vi "CAN Log File Data Write.vi"(5 "Size":string, 7 "Socket":i16, 8 "error in (no error)":errorcluster, 9 "With Column and CAN Data":string, 10 "Without Column and CAN Data":string, 11 "Byte Stream File in":refnum<file>) -> (0 "error out":errorcluster, 3 "Byte Stream File out":refnum<file>)   [LabVIEW 2023, in "LTT_TeststandSteptypes.lvlib"]
uses:
  LTT_TeststandSteptypes.lvlib
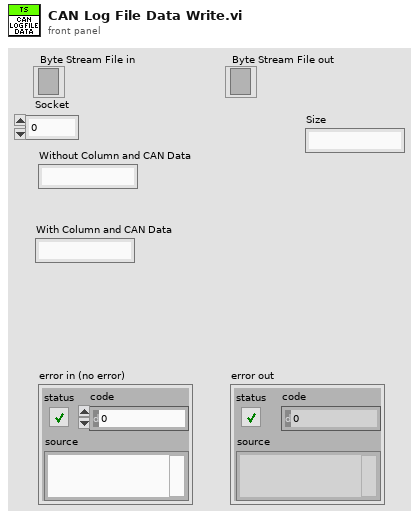
[diagram p1: front panel]
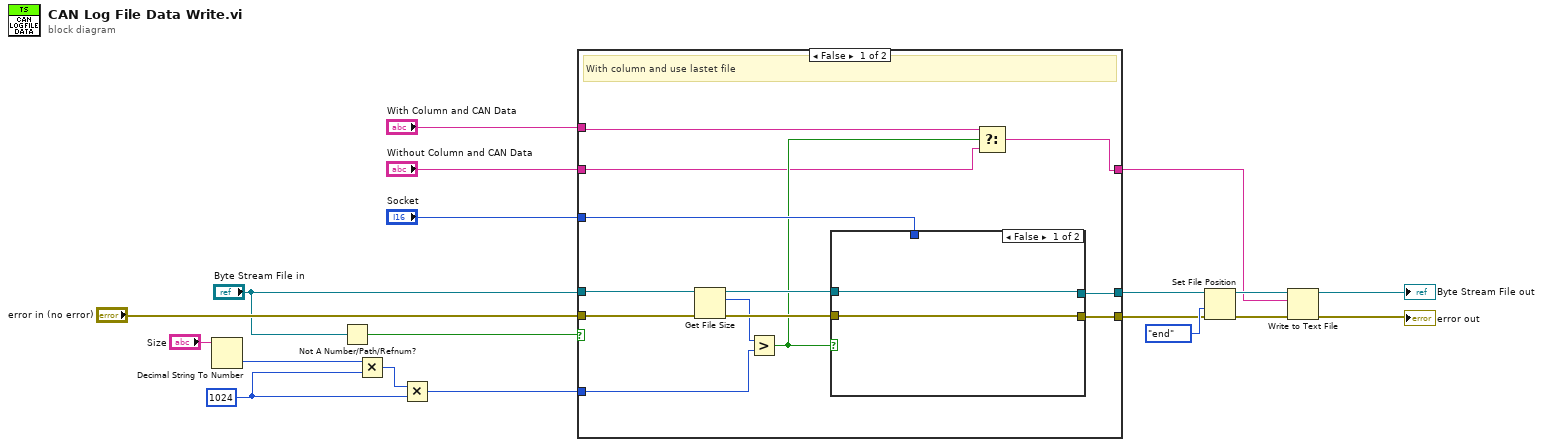
[diagram p0: block diagram]
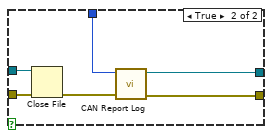
[diagram p2: hidden frame]
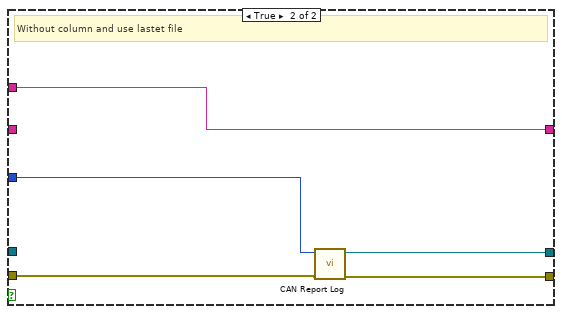
[diagram p3: hidden frame]
diagram:
  w5 = 1024 ("y")
  n1 = Decimal String To Number(string="Size") -> (number=w4:i32)  [unwired: 2 in, 1 out]
  n2 = Not A Number/Path/Refnum?(number/path/refnum="Byte Stream File in") -> (NaN/Path/Refnum?=w6:bool)
  n3 = Multiply(x=w4, y=w5) -> (x*y=w14:i32)
  n4 = Multiply(x=w14, y=w5) -> (x*y=w2:i32)
  n5 = case shown="False" w6 {
    tunnel: "error in (no error)" -> [w28 w45]
    tunnel: "Socket" -> [w32 w42]
    tunnel: "Byte Stream File in" -> [w29 _]
    tunnel: [w31 w44] -> w12
    tunnel: [w30 w43] -> w11
    tunnel: "With Column and CAN Data" -> [w22 w41]
    tunnel: "Without Column and CAN Data" -> [w21 _]
    tunnel: [w20 w41] -> w7
    tunnel: w2 -> [w25 _]
    frame False {
      # "With column and use lastet file"
      n6 = Get File Size(file=w29, error in=w28) -> (refnum out=w24:refnum<file>, size (in bytes)=w26:i64, 0:w27:errorcluster)
      n7 = Greater?(x=w26, y=w25) -> (0:w23:bool)
      n8 = case shown="False" w23 {
        tunnel: w32 -> [_ w40]
        tunnel: [w34 w39] -> w31
        tunnel: [w33 w38] -> w30
        tunnel: w27 -> [w33 w36]
        tunnel: w24 -> [w34 w35]
        frame False {
        }
        frame True {
          n9 = Close File(refnum=w35, error in=w36) -> (error out=w37:errorcluster)  [unwired: 1 out]
          n10 = call "CAN Report Log.vi"("error in (no error)"=w37, "Socket"=w40) -> ("error out"=w38:errorcluster, "refnum out"=w39:refnum<file>)  [unwired: 7 in, 1 out]
        }
      }
      n11 = Select(t=w22, s=w23, f=w21) -> (s? t:f=w20:string)
    }
    frame True {
      # "Without column and use lastet file"
      n12 = call "CAN Report Log.vi"("error in (no error)"=w45, "Socket"=w42) -> ("error out"=w43:errorcluster, "refnum out"=w44:refnum<file>)  [unwired: 7 in, 1 out]
    }
  }
  n13 = Set File Position(refnum=w12, from (0:start)=enum16{"start", "end", "current"}."end", error in=w11) -> (refnum out=w17:refnum<file>, error out=w18:errorcluster)  [unwired: 1 in]
  n14 = Write to Text File(file (use dialog)=w17, text=w7, error in=w18) -> (refnum out=→"Byte Stream File out":refnum<file>, error out=→"error out":errorcluster)  [unwired: 1 in, 1 out]
